vi "rotate.vi"() -> ()   [LabVIEW 2017]
uses:
  Control 1.ctl
panel:
  out "Numeric 3":sgl[][](array[numeric])
  out "Numeric 2":sgl[][](array[numeric])
  out "Numeric":sgl[][](array[numeric])
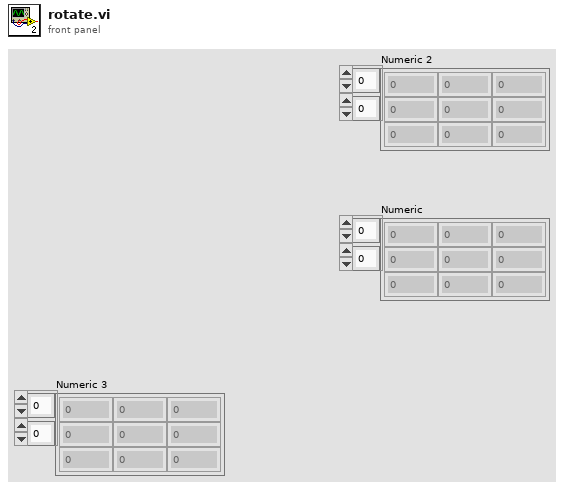
[diagram p1: front panel]
types:
  T1 = typedef "Control 1.ctl" = enum16{"1", "2", "3", "4", "5", "6", "7", "8", "9"}
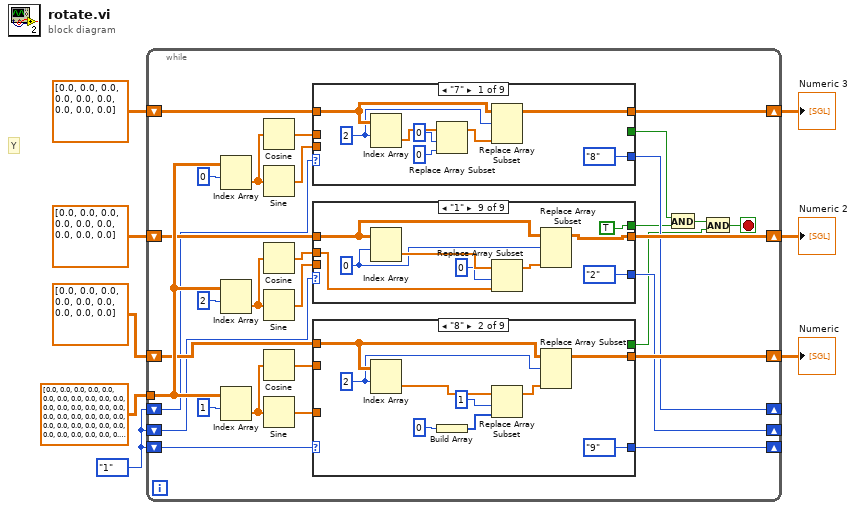
[diagram p0: block diagram]
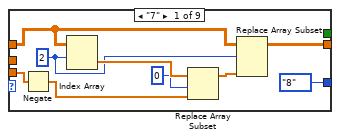
[diagram p2: hidden frame]
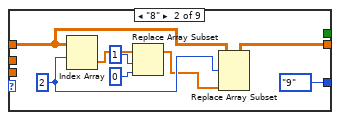
[diagram p3: hidden frame]
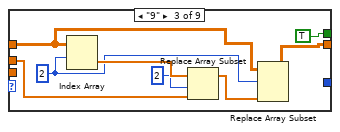
[diagram p4: hidden frame]
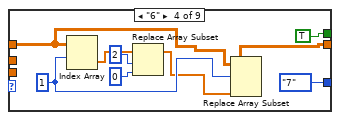
[diagram p5: hidden frame]
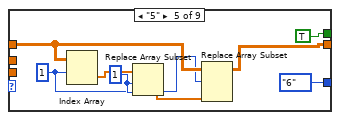
[diagram p6: hidden frame]
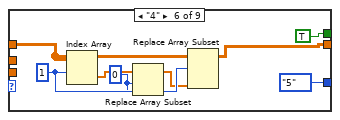
[diagram p7: hidden frame]
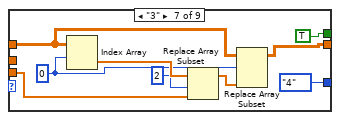
[diagram p8: hidden frame]
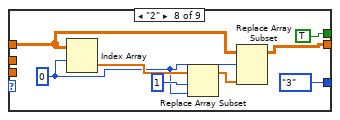
[diagram p9: hidden frame]
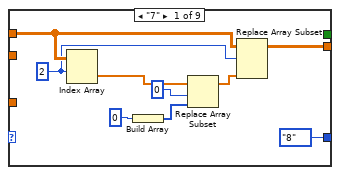
[diagram p10: hidden frame]
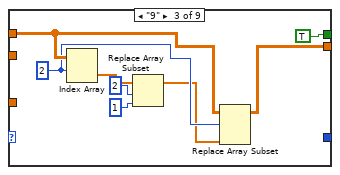
[diagram p11: hidden frame]
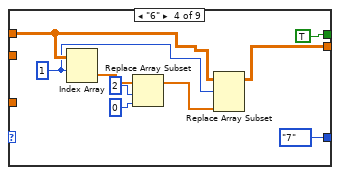
[diagram p12: hidden frame]
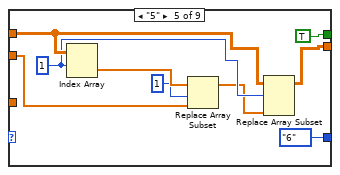
[diagram p13: hidden frame]
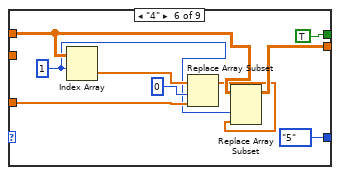
[diagram p14: hidden frame]
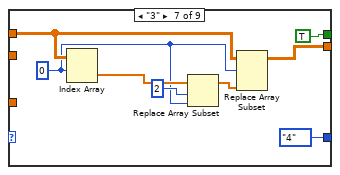
[diagram p15: hidden frame]
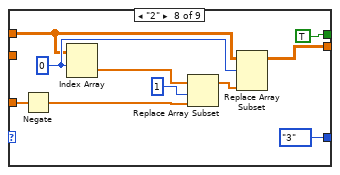
[diagram p16: hidden frame]
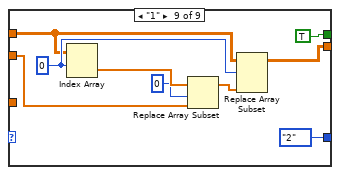
[diagram p17: hidden frame]
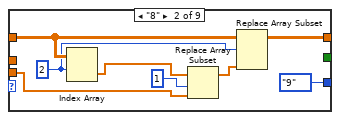
[diagram p18: hidden frame]
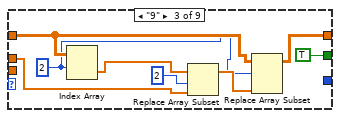
[diagram p19: hidden frame]
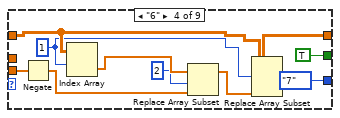
[diagram p20: hidden frame]
diagram:
  w4 = Control_1."1"
  # "Y"
  n1 = while {
    tunnel: sgl[][] [[0.0, 0.0, 0.0, 0.0, 0.0, 0.0], [0.0, 0.0, 0.0, 0.0, 0.0, 0.0], [0.0, 0.0, 0.0, 0.0, 0.0, 0.0], [0.0, 0.0, 0.0, 0.0, 0.0, 0.0], [0.0, 0.0, 0.0, 0.0, 0.0, 0.0], [0.0, 0.0, 0.0, 0.0, 0.0, 0.0]] -> [w38]
    shift-right: [w29] -> w1
    shift-left: sgl[][] [[0.0, 0.0, 0.0], [0.0, 0.0, 0.0], [0.0, 0.0, 0.0]] ("Numeric") -> [w30]
    shift-right: [w24] -> w2
    shift-left: sgl[][] [[0.0, 0.0, 0.0], [0.0, 0.0, 0.0], [0.0, 0.0, 0.0]] ("Numeric") -> [w25]
    shift-right: [w23] -> w3
    shift-left: sgl[][] [[0.0, 0.0, 0.0], [0.0, 0.0, 0.0], [0.0, 0.0, 0.0]] ("Numeric") -> [w26]
    shift-right: [w14] -> _
    shift-left: w4 -> [w17]
    shift-right: [w13] -> _
    shift-left: w4 -> [w16]
    shift-right: [w12] -> _
    shift-left: w4 -> [w15]
    stop <- w28 stop-if-true
    n2 = Index Array(array=w38, index (row)=0) -> (element=w34:sgl[])  [unwired: 1 in]
    n3 = Index Array(array=w38, index (row)=2) -> (element=w31:sgl[])  [unwired: 1 in]
    n4 = Index Array(array=w38, index (row)=1) -> (element=w32:sgl[])  [unwired: 1 in]
    n5 = Cosine(x=w34) -> (cos(x)=w20:sgl[])
    n6 = Sine(x=w34) -> (sin(x)=w33:sgl[])
    n7 = Cosine(x=w31) -> (cos(x)=w22:sgl[])
    n8 = Sine(x=w31) -> (sin(x)=w21:sgl[])
    n9 = Cosine(x=w32) -> (cos(x)=w18:sgl[])
    n10 = Sine(x=w32) -> (sin(x)=w19:sgl[])
    n11 = case shown="\"7\"" w17 {
      tunnel: w30 -> [w197 w206 w214 w221 w232 w241 w250 w259 w268]
      tunnel: w20 -> [_ _ w215 _ w234 _ _ _ _]
      tunnel: w33 -> [_ w207 _ w224 _ _ _ _ _]
      tunnel: [Control_1."8" Control_1."9" _ Control_1."7" Control_1."6" Control_1."5" Control_1."4" Control_1."3" Control_1."2"] -> w14
      tunnel: [w198 w205 w213 w222 w231 w238 w249 w258 w267] -> w29
      tunnel: [_ _ TRUE TRUE TRUE TRUE TRUE TRUE TRUE] -> w27
      frame "7" {
        w196 = 2 ("index (row)")
        n12 = Index Array(array=w197, index (row)=w196) -> (element=w201:sgl[])  [unwired: 1 in]
        n13 = Replace Array Subset(array=w201, new element=0, index=0 ("disabled index (col)")) -> (w195:sgl[])
        n14 = Replace Array Subset(array=w197, new element=w195, index (row)=w196) -> (w198:sgl[][])  [unwired: 1 in]
      }
      frame "8" {
        w204 = 2 ("index (row)")
        n15 = Index Array(array=w206, index (row)=w204) -> (element=w209:sgl[])  [unwired: 1 in]
        n16 = Replace Array Subset(array=w209, new element=w207, index=1 ("disabled index (col)")) -> (w203:sgl[])
        n17 = Replace Array Subset(array=w206, new element=w203, index (row)=w204) -> (w205:sgl[][])  [unwired: 1 in]
      }
      frame "9" {
        w211 = 2 ("index (row)")
        n18 = Index Array(array=w214, index (row)=w211) -> (element=w217:sgl[])  [unwired: 1 in]
        n19 = Replace Array Subset(array=w217, new element=w215, index=2 ("disabled index (col)")) -> (w212:sgl[])
        n20 = Replace Array Subset(array=w214, new element=w212, index (row)=w211) -> (w213:sgl[][])  [unwired: 1 in]
      }
      frame "6" {
        w220 = 1 ("index (row)")
        n21 = Negate(x=w224) -> (-x=w223:sgl[])
        n22 = Index Array(array=w221, index (row)=w220) -> (element=w227:sgl[])  [unwired: 1 in]
        n23 = Replace Array Subset(array=w227, new element=w223, index=2 ("disabled index (col)")) -> (w219:sgl[])
        n24 = Replace Array Subset(array=w221, new element=w219, index (row)=w220) -> (w222:sgl[][])  [unwired: 1 in]
      }
      frame "5" {
        w230 = 1 ("index (row)")
        n25 = Index Array(array=w232, index (row)=w230) -> (element=w236:sgl[])  [unwired: 1 in]
        n26 = Replace Array Subset(array=w236, new element=w234, index=1 ("disabled index (col)")) -> (w229:sgl[])
        n27 = Replace Array Subset(array=w232, new element=w229, index (row)=w230) -> (w231:sgl[][])  [unwired: 1 in]
      }
      frame "4" {
        w240 = 1 ("index (row)")
        n28 = Index Array(array=w241, index (row)=w240) -> (element=w245:sgl[])  [unwired: 1 in]
        n29 = Replace Array Subset(array=w245, new element=0, index=0 ("disabled index (col)")) -> (w239:sgl[])
        n30 = Replace Array Subset(array=w241, new element=w239, index (row)=w240) -> (w238:sgl[][])  [unwired: 1 in]
      }
      frame "3" {
        w252 = 0 ("index (row)")
        n31 = Index Array(array=w250, index (row)=w252) -> (element=w254:sgl[])  [unwired: 1 in]
        n32 = Replace Array Subset(array=w254, new element=0, index=2 ("disabled index (col)")) -> (w251:sgl[])
        n33 = Replace Array Subset(array=w250, new element=w251, index (row)=w252) -> (w249:sgl[][])  [unwired: 1 in]
      }
      frame "2" {
        w261 = 0 ("index (row)")
        n34 = Index Array(array=w259, index (row)=w261) -> (element=w263:sgl[])  [unwired: 1 in]
        n35 = Replace Array Subset(array=w263, new element=0, index=1 ("disabled index (col)")) -> (w260:sgl[])
        n36 = Replace Array Subset(array=w259, new element=w260, index (row)=w261) -> (w258:sgl[][])  [unwired: 1 in]
      }
      frame "1" {
        w270 = 0 ("index (row)")
        n37 = Index Array(array=w268, index (row)=w270) -> (element=w272:sgl[])  [unwired: 1 in]
        n38 = Replace Array Subset(array=w272, new element=1, index=0 ("disabled index (col)")) -> (w269:sgl[])
        n39 = Replace Array Subset(array=w268, new element=w269, index (row)=w270) -> (w267:sgl[][])  [unwired: 1 in]
      }
    }
    n40 = case shown="\"1\"" w16 {
      tunnel: w25 -> [w42 w50 w59 w66 w76 w84 w92 w102 w108]
      tunnel: w22 -> [_ _ w60 _ _ _ _ _ w111]
      tunnel: [Control_1."8" Control_1."9" _ Control_1."7" Control_1."6" Control_1."5" Control_1."4" Control_1."3" Control_1."2"] -> w13
      tunnel: [w41 w51 w58 w67 w75 w83 w91 w101 w109] -> w24
      tunnel: [_ _ TRUE TRUE TRUE TRUE TRUE TRUE TRUE] -> w11
      tunnel: w21 -> [w43 _ _ _ _ _ w89 _ _]
      frame "7" {
        w40 = 2 ("index (row)")
        n41 = Negate(x=w43) -> (-x=w44:sgl[])
        n42 = Index Array(array=w42, index (row)=w40) -> (element=w46:sgl[])  [unwired: 1 in]
        n43 = Replace Array Subset(array=w46, new element=w44, index=0 ("disabled index (col)")) -> (w39:sgl[])
        n44 = Replace Array Subset(array=w42, new element=w39, index (row)=w40) -> (w41:sgl[][])  [unwired: 1 in]
      }
      frame "8" {
        w49 = 2 ("index (row)")
        n45 = Index Array(array=w50, index (row)=w49) -> (element=w54:sgl[])  [unwired: 1 in]
        n46 = Replace Array Subset(array=w54, new element=0, index=1 ("disabled index (col)")) -> (w48:sgl[])
        n47 = Replace Array Subset(array=w50, new element=w48, index (row)=w49) -> (w51:sgl[][])  [unwired: 1 in]
      }
      frame "9" {
        w57 = 2 ("index (row)")
        n48 = Index Array(array=w59, index (row)=w57) -> (element=w62:sgl[])  [unwired: 1 in]
        n49 = Replace Array Subset(array=w62, new element=w60, index=2 ("disabled index (col)")) -> (w56:sgl[])
        n50 = Replace Array Subset(array=w59, new element=w56, index (row)=w57) -> (w58:sgl[][])  [unwired: 1 in]
      }
      frame "6" {
        w65 = 1 ("index (row)")
        n51 = Index Array(array=w66, index (row)=w65) -> (element=w71:sgl[])  [unwired: 1 in]
        n52 = Replace Array Subset(array=w71, new element=0 ("disabled index (col)"), index=2 ("disabled index (col)")) -> (w64:sgl[])
        n53 = Replace Array Subset(array=w66, new element=w64, index (row)=w65) -> (w67:sgl[][])  [unwired: 1 in]
      }
      frame "5" {
        w77 = 1 ("disabled index (col)")
        w74 = 1 ("index (row)")
        n54 = Index Array(array=w76, index (row)=w74) -> (element=w79:sgl[])  [unwired: 1 in]
        n55 = Replace Array Subset(array=w79, new element=w77, index=w77) -> (w73:sgl[])
        n56 = Replace Array Subset(array=w76, new element=w73, index (row)=w74) -> (w75:sgl[][])  [unwired: 1 in]
      }
      frame "4" {
        w81 = 0 ("disabled index (col)")
        w86 = 1 ("index (row)")
        n57 = Index Array(array=w84, index (row)=w86) -> (element=w87:sgl[])  [unwired: 1 in]
        n58 = Replace Array Subset(array=w87, new element=w81, index=w81) -> (w85:sgl[])
        n59 = Replace Array Subset(array=w84, new element=w85, index (row)=w86) -> (w83:sgl[][])  [unwired: 1 in]
      }
      frame "3" {
        w94 = 0 ("index (row)")
        n60 = Index Array(array=w92, index (row)=w94) -> (element=w96:sgl[])  [unwired: 1 in]
        n61 = Replace Array Subset(array=w96, new element=w89, index=2 ("disabled index (col)")) -> (w93:sgl[])
        n62 = Replace Array Subset(array=w92, new element=w93, index (row)=w94) -> (w91:sgl[][])  [unwired: 1 in]
      }
      frame "2" {
        w98 = 0 ("index (row)")
        n63 = Index Array(array=w102, index (row)=w98) -> (element=w104:sgl[])  [unwired: 1 in]
        n64 = Replace Array Subset(array=w104, new element=w98, index=1 ("index (row)")) -> (w103:sgl[])
        n65 = Replace Array Subset(array=w102, new element=w103, index (row)=w98) -> (w101:sgl[][])  [unwired: 1 in]
      }
      frame "1" {
        w106 = 0 ("index (row)")
        n66 = Index Array(array=w108, index (row)=w106) -> (element=w113:sgl[])  [unwired: 1 in]
        n67 = Replace Array Subset(array=w113, new element=w111, index=0 ("disabled index (col)")) -> (w107:sgl[])
        n68 = Replace Array Subset(array=w108, new element=w107, index (row)=w106) -> (w109:sgl[][])  [unwired: 1 in]
      }
    }
    n69 = case shown="\"8\"" w15 {
      tunnel: w26 -> [w117 w127 w135 w143 w152 w161 w171 w180 w189]
      tunnel: w18 -> [_ _ _ _ w155 _ _ _ w188]
      tunnel: [Control_1."8" Control_1."9" _ Control_1."7" Control_1."6" Control_1."5" Control_1."4" Control_1."3" Control_1."2"] -> w12
      tunnel: [w118 w126 w136 w144 w153 w162 w170 w179 w187] -> w23
      tunnel: [_ _ TRUE TRUE TRUE TRUE TRUE TRUE TRUE] -> w9
      tunnel: w19 -> [_ _ _ _ _ w163 _ w176 _]
      frame "7" {
        w116 = 2 ("index (row)")
        n70 = Index Array(array=w117, index (row)=w116) -> (element=w120:sgl[])  [unwired: 1 in]
        n71 = Build Array(0) -> (w122:i32[])
        n72 = Replace Array Subset(array=w120, new element=w122, index=0 ("disabled index (col)")) -> (w115:sgl[])
        n73 = Replace Array Subset(array=w117, new element=w115, index (row)=w116) -> (w118:sgl[][])  [unwired: 1 in]
      }
      frame "8" {
        w125 = 2 ("index (row)")
        n74 = Index Array(array=w127, index (row)=w125) -> (element=w129:sgl[])  [unwired: 1 in]
        n75 = Build Array(0) -> (w130:i32[])
        n76 = Replace Array Subset(array=w129, new element=w130, index=1 ("disabled index (col)")) -> (w124:sgl[])
        n77 = Replace Array Subset(array=w127, new element=w124, index (row)=w125) -> (w126:sgl[][])  [unwired: 1 in]
      }
      frame "9" {
        w134 = 2 ("index (row)")
        n78 = Index Array(array=w135, index (row)=w134) -> (element=w139:sgl[])  [unwired: 1 in]
        n79 = Replace Array Subset(array=w139, new element=1 ("disabled index (col)"), index=2 ("disabled index (col)")) -> (w133:sgl[])
        n80 = Replace Array Subset(array=w135, new element=w133, index (row)=w134) -> (w136:sgl[][])  [unwired: 1 in]
      }
      frame "6" {
        w142 = 1 ("index (row)")
        n81 = Index Array(array=w143, index (row)=w142) -> (element=w148:sgl[])  [unwired: 1 in]
        n82 = Replace Array Subset(array=w148, new element=0 ("disabled index (col)"), index=2 ("disabled index (col)")) -> (w141:sgl[])
        n83 = Replace Array Subset(array=w143, new element=w141, index (row)=w142) -> (w144:sgl[][])  [unwired: 1 in]
      }
      frame "5" {
        w151 = 1 ("index (row)")
        n84 = Index Array(array=w152, index (row)=w151) -> (element=w157:sgl[])  [unwired: 1 in]
        n85 = Replace Array Subset(array=w157, new element=w155, index=1 ("disabled index (col)")) -> (w150:sgl[])
        n86 = Replace Array Subset(array=w152, new element=w150, index (row)=w151) -> (w153:sgl[][])  [unwired: 1 in]
      }
      frame "4" {
        w160 = 1 ("index (row)")
        n87 = Index Array(array=w161, index (row)=w160) -> (element=w166:sgl[])  [unwired: 1 in]
        n88 = Replace Array Subset(array=w166, new element=w163, index=0 ("disabled index (col)")) -> (w159:sgl[])
        n89 = Replace Array Subset(array=w161, new element=w159, index (col)=w160) -> (w162:sgl[][])  [unwired: 1 in]
      }
      frame "3" {
        w168 = 0 ("index (row)")
        n90 = Index Array(array=w171, index (row)=w168) -> (element=w174:sgl[])  [unwired: 1 in]
        n91 = Replace Array Subset(array=w174, new element=w168, index=2 ("disabled index (col)")) -> (w172:sgl[])
        n92 = Replace Array Subset(array=w171, new element=w172, index (row)=w168) -> (w170:sgl[][])  [unwired: 1 in]
      }
      frame "2" {
        w182 = 0 ("index (row)")
        n93 = Negate(x=w176) -> (-x=w177:sgl[])
        n94 = Index Array(array=w180, index (row)=w182) -> (element=w184:sgl[])  [unwired: 1 in]
        n95 = Replace Array Subset(array=w184, new element=w177, index=1 ("disabled index (col)")) -> (w181:sgl[])
        n96 = Replace Array Subset(array=w180, new element=w181, index (row)=w182) -> (w179:sgl[][])  [unwired: 1 in]
      }
      frame "1" {
        w191 = 0 ("index (row)")
        n97 = Index Array(array=w189, index (row)=w191) -> (element=w193:sgl[])  [unwired: 1 in]
        n98 = Replace Array Subset(array=w193, new element=w188, index=0 ("disabled index (col)")) -> (w190:sgl[])
        n99 = Replace Array Subset(array=w189, new element=w190, index (row)=w191) -> (w187:sgl[][])  [unwired: 1 in]
      }
    }
    n100 = And(x=w27, y=w11) -> (x .and. y?=w10:bool)
    n101 = And(x=w10, y=w9) -> (x .and. y?=w28:bool)
  }
  "Numeric" <- w3
  "Numeric 2" <- w2
  "Numeric 3" <- w1
